vi "_Parse Limit Check Array Result.vi"(0 "error in (no error)":errorcluster, 2 "Input String":string, 3 "VISA resource name":refnum<visa-resource-name>, 4 "Out of tolerance? (F)":bool) -> (6 "Out Of Tolerance":i32, 7 "error out":errorcluster, 8 "Results":i32[](array[numeric]), 9 "Reliability":i32, 10 "VISA resource name out":refnum<visa-resource-name>)   [LabVIEW 2020, in "Rohde&Schwarz CMWXP NR FR1 Measurement.lvlib"]
uses:
  <instrlib>/Rohde&Schwarz CMWXP NR FR1 Measurement/Rohde&Schwarz CMWXP NR FR1 Measurement.lvlib
  <instrlib>/Rohde&Schwarz CMWXP NR FR1 Measurement/Private/rsidr_core.llb/rsidr_core.lvlib
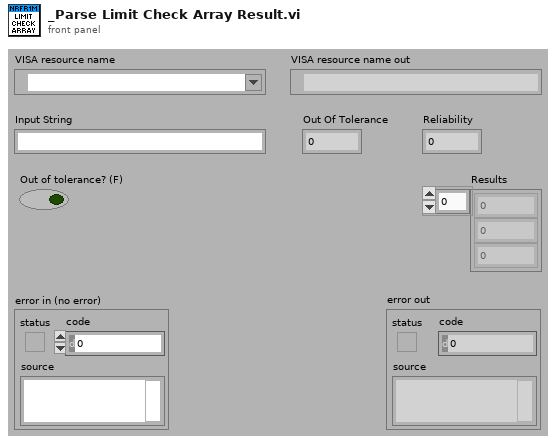
[diagram p1: front panel]
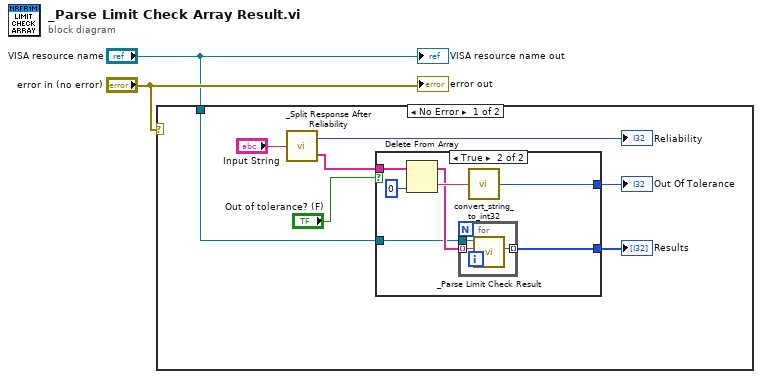
[diagram p0: block diagram]
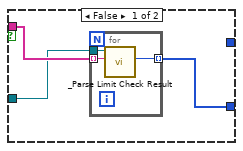
[diagram p2: hidden frame]
diagram:
  n1 = case shown="No Error" "error in (no error)" {
    tunnel: "VISA resource name" -> [w4 _]
    frame No Error {
      n2 = call <instrlib>:"_Split Response After Reliability.vi"("Input String"="Input String") -> ("Response out"=w7:string[], "Reliability out"=→"Reliability":i32)
      n3 = case shown="True" "Out of tolerance? (F)" {
        tunnel: w7 -> [w12 w22]
        tunnel: [w11 w16] -> w6
        tunnel: w4 -> [w10 w18]
        tunnel: [_ w17] -> w3
        frame False {
          n4 = for {
            tunnel: [w15] -> w11 mode=indexing
            tunnel: w12 -> [w14] mode=indexing
            tunnel: w10 -> [w13]
            n5 = call <instrlib>:"_Parse Limit Check Result.vi"("String Value In"=w14, "VISA resource name"=w13) -> ("Limit Check Value"=w15:i32)  [unwired: 7 in, 2 out]
          }
        }
        frame True {
          n6 = Delete From Array(array=w22, index=0) -> (deleted portion=w20:string, array with subset deleted=w19:string[])  [unwired: 1 in]
          n7 = for {
            tunnel: [w25] -> w16 mode=indexing
            tunnel: w19 -> [w24] mode=indexing
            tunnel: w18 -> [w23]
            n8 = call <instrlib>:"_Parse Limit Check Result.vi"("String Value In"=w24, "VISA resource name"=w23) -> ("Limit Check Value"=w25:i32)  [unwired: 7 in, 2 out]
          }
          n9 = call <instrlib>:"convert_string_to_int32.vi"("String in"=w20) -> ("int32 value out"=w17:i32)  [unwired: 4 in]
        }
      }
      "Results" <- w6
      "Out Of Tolerance" <- w3
    }
    frame Error {
    }
  }
  "VISA resource name out" <- "VISA resource name"
  "error out" <- "error in (no error)"
